vi "Error Test Start Bit Value.vi"(6 "error text in":string, 8 "error in":errorcluster, 9 "start bit":i32) -> (0 "error out":errorcluster)   [LabVIEW 2020]
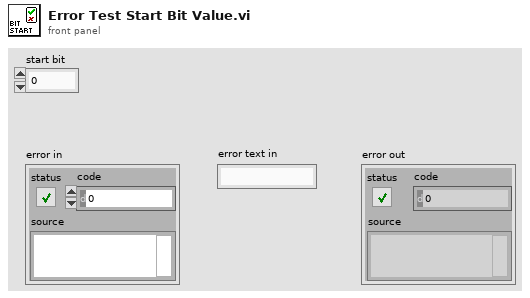
[diagram p1: front panel]
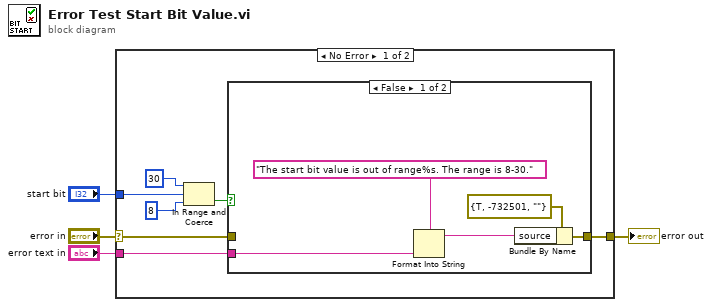
[diagram p0: block diagram]
diagram:
  n1 = case shown="No Error" "error in" {
    selector: "error in" -> [w10 w18]
    tunnel: [w9 w18] -> w3
    tunnel: "start bit" -> [w11 _]
    tunnel: "error text in" -> [w8 _]
    frame No Error {
      n2 = In Range and Coerce(upper limit=30 ("lower limit"), x=w11, lower limit=8) -> (In Range?=w5:bool)  [unwired: 1 out]
      n3 = case shown="False" w5 {
        tunnel: w10 -> [_ w17]
        tunnel: [w16 w17] -> w9
        tunnel: w8 -> [w13 _]
        frame False {
          n4 = Format Into String(format string="The start bit value is out of range%s. The range is 8-30." ("source"), w13) -> (resulting string=w15:string)  [unwired: 2 in, 1 out]
          n5 = Bundle By Name(cluster=errorcluster {"status"=TRUE, "code"=-732501, "source"=""} ("error constant"), "source"=w15) -> (w16:errorcluster)
        }
        frame True {
        }
      }
    }
    frame Error {
    }
  }
  "error out" <- w3
